vi "testPositionSDO6064.vi"() -> ()   [LabVIEW 2013]
uses:
  <vilib>/CANopenLib/CANOPEN.llb/CANopen BaudRate.ctl
  <vilib>/CANopenLib/CANOPEN.llb/CANopen Interface Create.vi
  <vilib>/CANopenLib/CANOPEN.llb/CANopen SDO Create.vi
  <vilib>/CANopenLib/CANOPEN.llb/CANopen SDO Close.vi
  <vilib>/CANopenLib/CANOPEN.llb/CANopen Interface Close.vi
  <vilib>/CANopenLib/CANOPEN.llb/CANopen SDO Read [I32].vi
panel:
  in  "Stopp":bool
  out "I32 data":i32
  # "Liest den Positionswert mit dem Canobjekt 6064h"
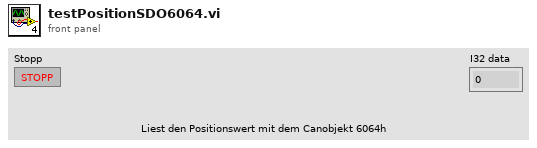
[diagram p1: front panel]
types:
  T1 = typedef "CANopen BaudRate.ctl" = u32
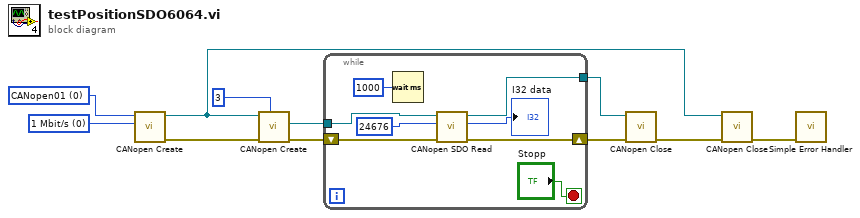
[diagram p0: block diagram]
diagram:
  w10 = T1 0 items=["1 Mbit/s"=0, "800 kbit/s"=1, "500 kbit/s"=2, "250 kbit/s"=3, "125 kbit/s"=4, "50 kbit/s"=6, "20 kbit/s"=7, "10 kbit/s"=8] ("baud rate")
  w11 = u32 0 items=["CANopen01", "CANopen02", "CANopen03", "CANopen04", "CANopen05", "CANopen06", "CANopen07", "CANopen08", "CANopen09", "CANopen10", "CANopen11", "CANopen12", "CANopen13", "CANopen14", "CANopen15", "CANopen16", "CANopen17", "CANopen18", "CANopen19", "CANopen20", "CANopen21", "CANopen22", "CANopen23", "CANopen24", "CANopen25", "CANopen26", "CANopen27", "CANopen28", "CANopen29", "CANopen30", "CANopen31", "CANopen32"] ("interface name")
  n1 = call-poly <vilib>:"CANopen Create.vi"("baud rate"=w10, "interface name"=w11) -> ("error out"=w9:errorcluster, "interface object out"=w3:refnum<k20>)  [unwired: 8 in]
  n2 = call-poly <vilib>:"CANopen Create.vi"("node-ID"=u8 3, "error in (no error)"=w9, "interface object in"=w3) -> ("error out"=w7:errorcluster, "SDO object out"=w8:refnum<k20>)  [unwired: 6 in, 1 out]
  n3 = while {
    tunnel: w8 -> [w19]
    tunnel: [w15] -> w5
    shift-right: [w16] -> w6
    shift-left: w7 -> [w17]
    stop <- "Stopp" stop-if-true
    n4 = Wait (ms)(milliseconds to wait=u32 1000 ("Zu wartende ms")) -> ()  [unwired: 1 out]
    n5 = call-poly <vilib>:"CANopen SDO Read.vi"("error in (no error)"=w17, "object index"=u16 24676, "SDO object in"=w19) -> ("error out"=w16:errorcluster, "I32 data"=→"I32 data":i32, "SDO object out"=w15:refnum<k20>)  [unwired: 5 in, 1 out]
  }
  n6 = call-poly <vilib>:"CANopen Close.vi"("error in (no error)"=w6, "SDO object in"=w5) -> ("error out"=w4:errorcluster)  [unwired: 9 in]
  n7 = call-poly <vilib>:"CANopen Close.vi"("error in (no error)"=w4, "interface object in"=w3) -> ("error out"=w2:errorcluster)  [unwired: 9 in]
  n8 = call <vilib>:"Simple Error Handler.vi"("error in (no error)"=w2) -> ()  [unwired: 4 in, 5 out]
